vi "Variant.vi"(4 "Value":T1=variant(timestamp timestamp(0 s since 1904-01-01))) -> (1 "Constant":refnum<class "Const_Variant.lvclass">)   [LabVIEW 2021, in "Const_Variant.lvclass"]
uses:
  Const_Variant.lvclass
  Type.ctl
  Const_Variant.lvclass/Const_Variant.ctl
  Properties/Write Value.vi
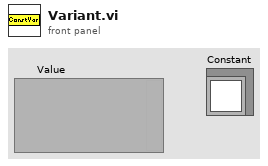
[diagram p1: front panel]
types:
  T1 = typedef "Const_Variant.lvclass/Type.ctl" = variant
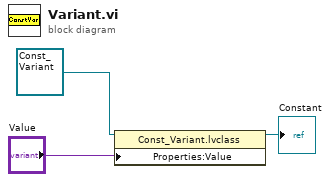
[diagram p0: block diagram]
diagram:
  n1 = property class="Const_Variant.lvclass"(reference=refnum<class "Const_Variant.lvclass"> refnum ("Constants.lvlib:Numeric.lvclass"), "Properties:Value"="Value") -> (reference out=→"Constant":refnum<class "Const_Variant.lvclass">)  [unwired: 1 in, 1 out]
